vi "Relocate Files.vi"(10 "Paths in":path[](array[path]), 11 "Working Folder":path) -> (1 "Files to delete":path[](array[path]), 2 "Paths out":path[](array[path]))   [LabVIEW 2018]
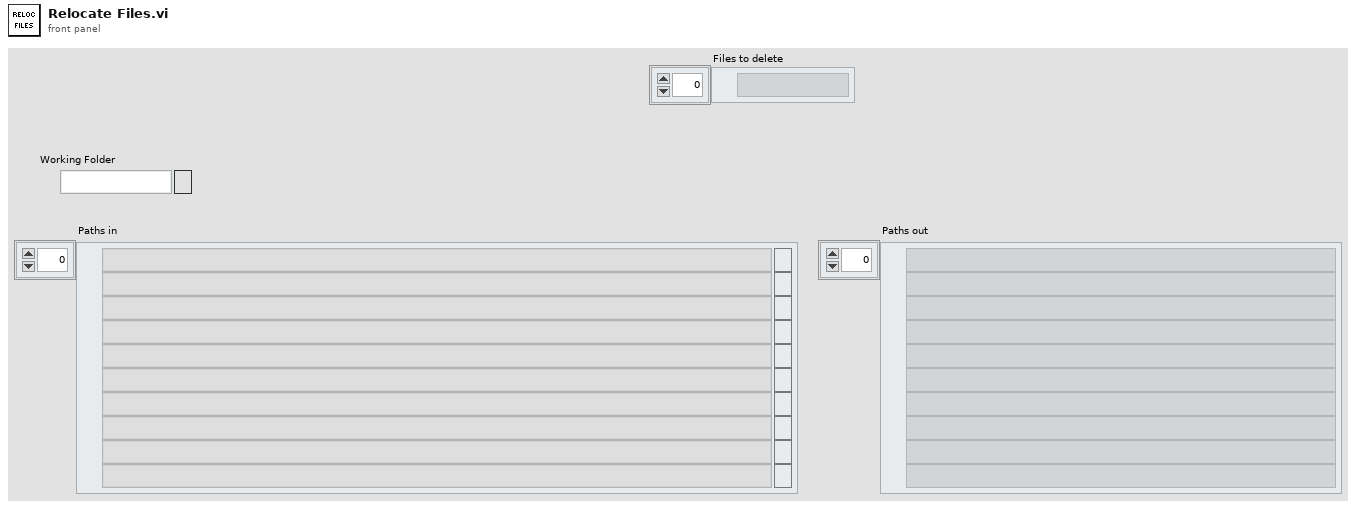
[diagram p1: front panel]
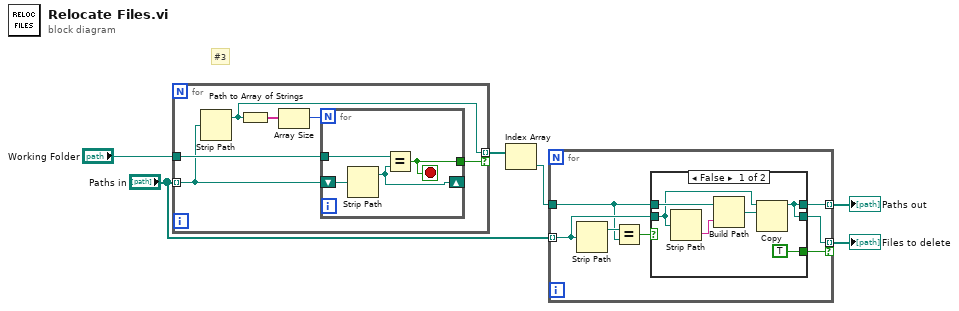
[diagram p0: block diagram]
diagram:
  # "#3"
  n1 = for {
    tunnel: "Paths in" -> [w9] mode=indexing
    tunnel: "Working Folder" -> [w12]
    tunnel: [w8] -> w5 mode=indexing if=w7
    n2 = Strip Path(path=w9) -> (stripped path=w8:path)  [unwired: 1 out]
    n3 = Path to Array of Strings(0:w8) -> (2:w11:string[])  [unwired: 1 out]
    n4 = Array Size(array=w11) -> (size(s)=w10:i32)
    n5 = for {
      N: w10 -> [_]
      tunnel: w12 -> [w15]
      tunnel: [w14] -> w7
      shift-right: [w13] -> _
      shift-left: w9 -> [w16]
      stop <- w14 stop-if-true
      n6 = Strip Path(path=w16) -> (stripped path=w13:path)  [unwired: 1 out]
      n7 = Equal?(x=w15, y=w13) -> (x = y?=w14:bool)
    }
  }
  n8 = Index Array(array=w5) -> (element=w3:path)  [unwired: 1 in]
  n9 = for {
    tunnel: "Paths in" -> [w20] mode=indexing
    tunnel: w3 -> [w19]
    tunnel: [w21] -> w1 mode=indexing
    tunnel: [w18] -> w2 mode=indexing if=w17
    n10 = Strip Path(path=w20) -> (stripped path=w23:path)  [unwired: 1 out]
    n11 = Equal?(x=w23, y=w19) -> (x = y?=w22:bool)
    n12 = case shown="False" w22 {
      tunnel: [w26 w30] -> w21
      tunnel: w20 -> [w24 w30]
      tunnel: w19 -> [w29 _]
      tunnel: [w26 _] -> w18
      tunnel: [TRUE _] -> w17
      frame False {
        n13 = Strip Path(path=w24) -> (name=w28:string)  [unwired: 1 out]
        n14 = Build Path(base path=w29, name or relative path=w28) -> (appended path=w27:path)
        n15 = Copy(10:w27, 11:w24) -> (3:w26:path)  [unwired: 3 in, 2 out]
      }
      frame True {
      }
    }
  }
  "Paths out" <- w1
  "Files to delete" <- w2
